vi "PH_SHS_Analysis_Calibrator.reset Attributes.vi"(0 "i ref in":refnum<vi>, 5 "error in (no error)":errorcluster) -> (14 "i ref out":refnum<vi>, 19 "error out":errorcluster)   [LabVIEW 2014, in "PH_SHS_Analysis_Calibrator.lvlib"]
doc: "This VI resets the attributes in case of a selecting another cam or canceling the calibration procedure, e.g.."
uses:
  PH_SHS_Analysis_Calibrator.lvlib
  CSlibraries-extern/shs/SHS_Common/SHSReference.ctl
  CSlibraries-extern/shs/SHS_Common/ReferencePoint.ctl
  CSlibraries-extern/shs/SHS_Common/Rectangle.ctl
  CSlibraries-extern/shs/SHS_Common/Point.ctl
  PH_Basics/PH_Common/PH_Common.lvlib
  CSlibraries-extern/shs/SHS_Common/SHS_Common.lvlib
  PH_Basics/PH_Img_BaseClass/PH_Img_BaseClass.lvlib
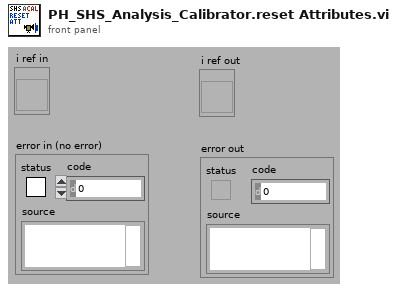
[diagram p1: front panel]
types:
  T1 = cluster{"Cam ID":string, "Gain":dbl, "Brightness":dbl, "Shutter":dbl, "Cam Error":bool, "Mode":i32}
  T2 = typedef "PH_SHS_Analysis_Calibrator.lvlib/PH_SHS_Analysis_Calibrator.i attribute.ctl" = cluster{"GUI Refs":cluster{"Available Cams":refnum<vi>, "OK":refnum<vi>, "Skip":refnum<vi>, "Repeat":refnum<vi>, "Cancel":refnum<vi>, "Dialog":refnum<vi>, "Enough Images?":refnum<vi>}, "Cam instances":string[], "Status":cluster{"#":i32, "Data calculated":bool, "Wanted #":i32}, "IMAQ Image Array":T3[], "Pixel Size [µm]":dbl, "MLA Pitch [µm]":dbl, "Method":enum16{"automatic", "manual"}, "Enough Images?":bool, "SHS Reference Result":T4, "Calculation Error":errorcluster}
  T3 = typedef "IMAQ Image.ctl" = refnum<image>
  T4 = typedef "SHS_Common.lvlib/SHSReference.ctl" = cluster{"Reference":T5[][], "Lens Array Pitch [px]":dbl}
  T5 = typedef "SHS_Common.lvlib/ReferencePoint.ctl" = cluster{"Rect":T6, "Point":T7}
  T6 = typedef "SHS_Common.lvlib/Rectangle.ctl" = cluster{"Left":i32, "Top":i32, "Right":i32, "Bottom":i32}
  T7 = typedef "SHS_Common.lvlib/Point.ctl" = cluster{"x":dbl, "y":dbl, "valid?":bool, "weight":dbl}
  T8 = typedef "PH_Img_BaseClass.lvlib/PH_Img_BaseClass.i attribute.ctl" = cluster{"GUI Refs":T9, "Timeout Image [ms]":i32, "Default Periodic Period [ms]":i32, "Camera":cluster{"Instancename":string, "Notifier":refnum<notifier>}, "Palette":T10, "Cam Settings":cluster{"Cam ID":string, "Gain":dbl, "Brightness":dbl, "Shutter":dbl, "Cam Info Failure":bool, "Mode":i32}}
  T9 = typedef "PH_Img_BaseClass.lvlib/PH_Img_BaseClass.GUI Refs.ctl" = cluster{"Timeout":refnum<vi>, "Image":refnum<vi>, "Palette":refnum<vi>, "Timeout Set":refnum<vi>}
  T10 = typedef "PH_Img_BaseClass.lvlib/PH_Img_BaseClass.Palette.ctl" = i32
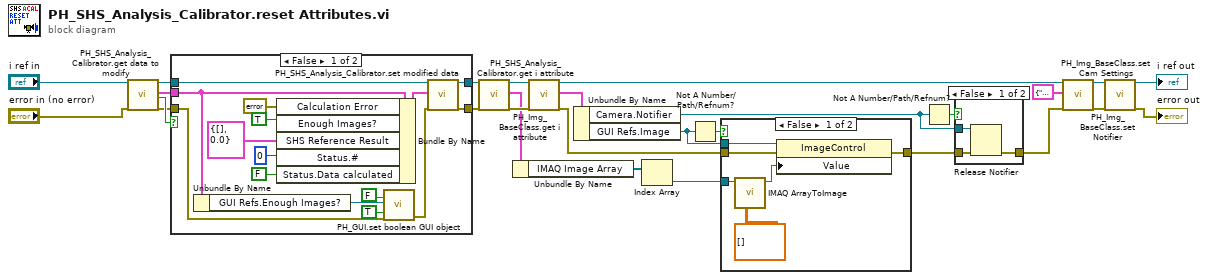
[diagram p0: block diagram]
diagram:
  n1 = call "PH_SHS_Analysis_Calibrator.get data to modify.vi"("i ref in"="i ref in", "error in (no error)"="error in (no error)") -> ("i ref out"=w22:refnum<vi>, "i attribute"=w24:T2, "timed out"=w25:bool, "error out"=w23:errorcluster)  [unwired: 14 in]
  n2 = case shown="False" w25 {
    tunnel: w22 -> [w42 w44]
    tunnel: w23 -> [w37 w43]
    tunnel: [w41 w44] -> w16
    tunnel: [w40 w43] -> w19
    tunnel: w24 -> [w38 _]
    frame False {
      n3 = Unbundle By Name(w38) -> ("GUI Refs.Enough Images?"=w34:refnum<vi>)
      n4 = Bundle By Name(cluster=w38, "Calculation Error"=errorcluster {"status"=FALSE, "code"=0, "source"=""}, "Enough Images?"=TRUE, "SHS Reference Result"=T4 {"Reference"=[], "Lens Array Pitch [px]"=0.0}, "Status.#"=0 ("Dark Pics.#"), "Status.Data calculated"=FALSE ("Dark Pics.BI taken")) -> (w39:T2)
      n5 = call "PH_GUI.set boolean GUI object.vi"("Visible (true)"=FALSE, "Boolean Knob GUI Ref"=w34, "Value"=TRUE, "error in (no error)"=w37) -> ("error out"=w28:errorcluster)  [unwired: 15 in]
      n6 = call "PH_SHS_Analysis_Calibrator.set modified data.vi"("i ref in"=w42, "i attribute"=w39, "error in (no error)"=w28) -> ("i ref out"=w41:refnum<vi>, "error out"=w40:errorcluster)  [unwired: 15 in]
    }
    frame True {
    }
  }
  n7 = call "PH_SHS_Analysis_Calibrator.get i attribute.vi"("i ref in"=w16, "error in (no error)"=w19) -> ("i ref out"=w15:refnum<vi>, "i attribute"=w10:T2, "error out"=w18:errorcluster)  [unwired: 15 in]
  n8 = Unbundle By Name(w10) -> ("IMAQ Image Array"=w9:T3[])
  n9 = call "PH_Img_BaseClass.get i attribute.vi"("i ref in"=w15, "error in (no error)"=w18) -> ("i ref out"=w14:refnum<vi>, "i attribute"=w11:T8, "error out"=w17:errorcluster)  [unwired: 15 in]
  n10 = Unbundle By Name(w11) -> ("Camera.Notifier"=w4:refnum<notifier>, "GUI Refs.Image"=w6:refnum<vi>)
  n11 = Index Array(array=w9) -> (element=w8:T3)  [unwired: 1 in]
  n12 = Not A Number/Path/Refnum?(number/path/refnum=w6) -> (NaN/Path/Refnum?=w7:bool)
  n13 = case shown="False" w7 {
    tunnel: w6 -> [w50 _]
    tunnel: w17 -> [w49 w51]
    tunnel: [w48 w51] -> w3
    tunnel: w8 -> [w46 _]
    frame False {
      n14 = call "IMAQ ArrayToImage"("Image Pixels (Float)"=sgl[][] [], "Image"=w46) -> ("Image Out"=w47:T3)  [unwired: 8 in, 1 out]
      n15 = property class="ImageControl"(reference=w50, error in=w49, "Value"=w47) -> (error out=w48:errorcluster)  [unwired: 1 out]
    }
    frame True {
    }
  }
  n16 = Not A Number/Path/Refnum?(number/path/refnum=w4) -> (NaN/Path/Refnum?=w5:bool)
  n17 = case shown="False" w5 {
    tunnel: w4 -> [w54 _]
    tunnel: w3 -> [w53 w55]
    tunnel: [w52 w55] -> w2
    frame False {
      n18 = Release Notifier(notifier=w54, error in (no error)=w53) -> (error out=w52:errorcluster)  [unwired: 1 in, 2 out]
    }
    frame True {
    }
  }
  n19 = call "PH_Img_BaseClass.set Cam Settings.vi"("i ref in"=w14, "Cam Settings"=T1 {"Cam ID"="N/A", "Gain"=nan, "Brightness"=nan, "Shutter"=nan, "Cam Error"=TRUE, "Mode"=-1}, "error in (no error)"=w2) -> ("i ref out"=w13:refnum<vi>, "error out"=w20:errorcluster)  [unwired: 15 in]
  n20 = call "PH_Img_BaseClass.set Notifier.vi"("i ref in"=w13, "error in"=w20) -> ("i ref out"=→"i ref out":refnum<vi>, "error out"=→"error out":errorcluster)  [unwired: 16 in]
